vi "Is VI Running.vi"(8 "error in (no error)":errorcluster, 11 "VI in":refnum<vi>) -> (0 "error out":errorcluster, 1 "VI Not Running":bool, 2 "VI Running":bool, 3 "VI out":refnum<vi>)   [LabVIEW 2023]
doc: "Returns True if referenced VI is running or running top level.\n\n12-12-15 added check for valid input reference, since if the VI is removed from memory it won't be a valid ref here, which will generate an error at property node. This would generate a \"Bad\" exe state, and the function would still work. ut this is cleaner and avoids an error condition.\n\nVI Not Running will be true ONLY IF the input VI Ref is valid."
panel:
  out "Valid VI ref?":bool
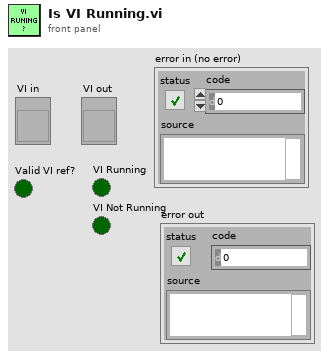
[diagram p1: front panel]
types:
  T1 = enum32{"Bad", "Idle", "Run top level", "Running"}
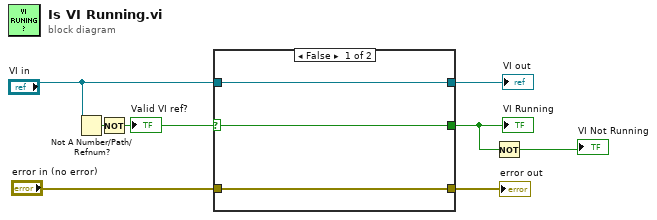
[diagram p0: block diagram]
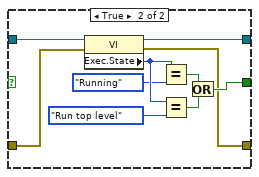
[diagram p2: hidden frame]
diagram:
  n1 = Not A Number/Path/Refnum?(number/path/refnum="VI in") -> (NaN/Path/Refnum?=w6:bool)
  n2 = Not(x=w6) -> (.not. x?=w2:bool)
  "Valid VI ref?" <- w2
  n3 = case shown="False" w2 {
    selector: w2 -> [w10 _]
    tunnel: [w10 w21] -> w3
    tunnel: [w11 w16] -> w8
    tunnel: "VI in" -> [w11 w14]
    tunnel: "error in (no error)" -> [w9 w13]
    tunnel: [w9 w12] -> w4
    frame False {
    }
    frame True {
      n4 = property class="VI"(reference=w14, error in=w13) -> (reference out=w16:refnum<vi>, error out=w12:errorcluster, "Exec.State"=w18:T1)
      n5 = Equal?(x=w18, y=T1."Running" ("Execution:State")) -> (x = y?=w20:bool)
      n6 = Equal?(x=w18, y=T1."Run top level" ("Execution:State")) -> (x = y?=w19:bool)
      n7 = Or(x=w20, y=w19) -> (x .or. y?=w21:bool)
    }
  }
  "VI Running" <- w3
  "VI out" <- w8
  "error out" <- w4
  n8 = Not(x=w3) -> (.not. x?=→"VI Not Running":bool)
